vi "主页面.vi"() -> ()   [LabVIEW 2018]
uses:
  Global_Variable/A131258.vi
panel:
  out "8MPa正逆向差值":dbl format="%#.3g"
  out "压销力":bool
  out "内泄露":bool
  out "力特性":bool
  out "回正率":dbl format="%#.3g"
  out "右滞后最小值":dbl format="%#.3g"
  out "右滞后最大值":dbl format="%#.3g"
  out "左滞后最小值":dbl format="%#.3g"
  out "左滞后最大值":dbl format="%#.3g"
  out "力特性":cluster{dbl[], dbl[]}[](graph)
  out "布尔":bool
  out "压销力(N)":dbl format="%#.3g"
  out "右内泄露值(L)":dbl format="%#.3g"
  out "左内泄露值(L)":dbl format="%#.3g"
  out "1MPa逆向最大扭矩":dbl format="%#.3g"
  out "1MPa正向最大扭矩":dbl format="%#.3g"
  out "全曲线对称性":dbl format="%#.3g"
  out "5MPa对称性":dbl format="%#.3g"
  out "1MPa对称性":dbl format="%#.3g"
  out "8MPa逆向最大扭矩":dbl format="%#.3g"
  out "8MPa正向最大扭矩":dbl format="%#.3g"
  out "5MPa逆向最大扭矩":dbl format="%#.3g"
  out "5MPa正向最大扭矩":dbl format="%#.3g"
  out "3MPa逆向最大扭矩":dbl format="%#.3g"
  out "3MPa正向最大扭矩":dbl format="%#.3g"
  out "逆向最大油压":dbl format="%#.3g"
  out "正向最大油压":dbl format="%#.3g"
  out "逆向最大扭矩":dbl format="%#.3g"
  out "正向最大扭矩":dbl format="%#.3g"
  in  "停止":bool
  # "调阀台"
  # "-10    -9     -8     -7     -6      -5    -4      -3     -2     -1       0      1       2      3       4       5      6      7      8      9       10"
  # "9"
  # "8"
  # "7"
  # "6"
  # "5"
  # "4"
  # "3"
  # "2"
  # "1"
  # "0"
  # "-10    -9     -8     -7     -6      -5    -4      -3     -2     -1       0      1       2      3       4       5      6      7      8      9       10"
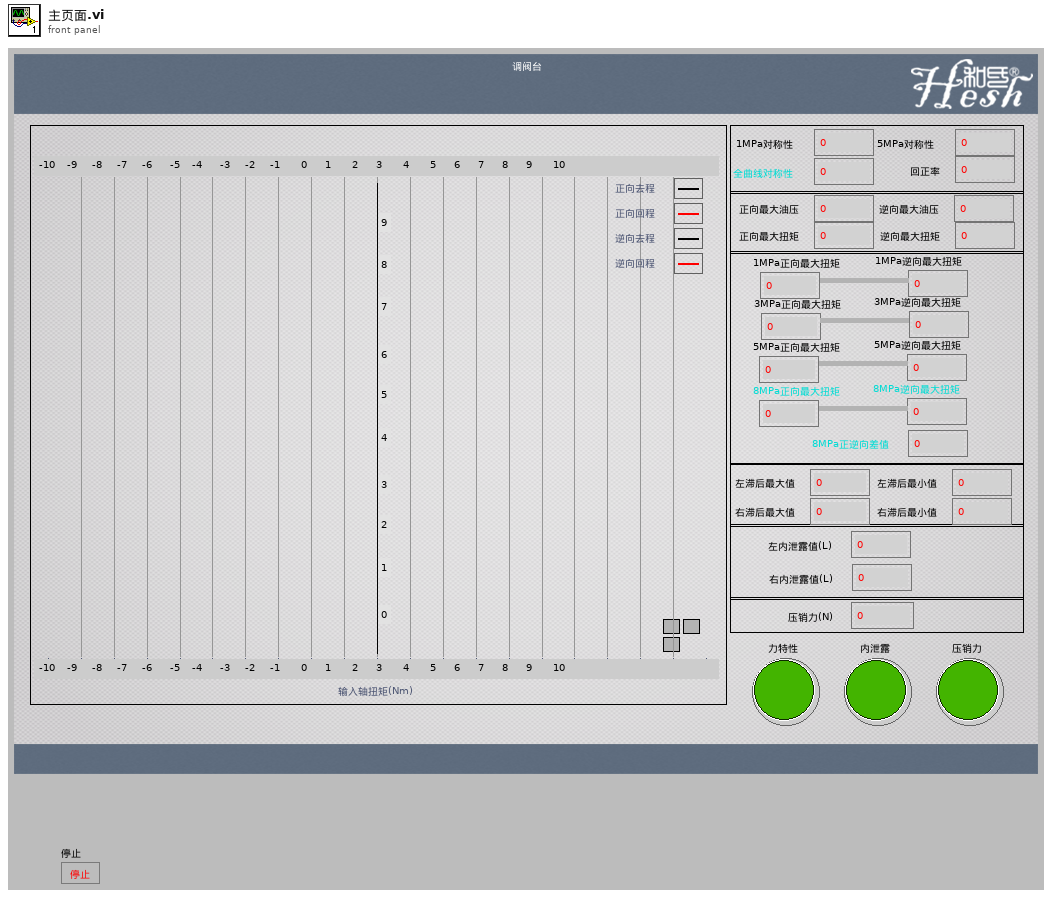
[diagram p1: front panel]
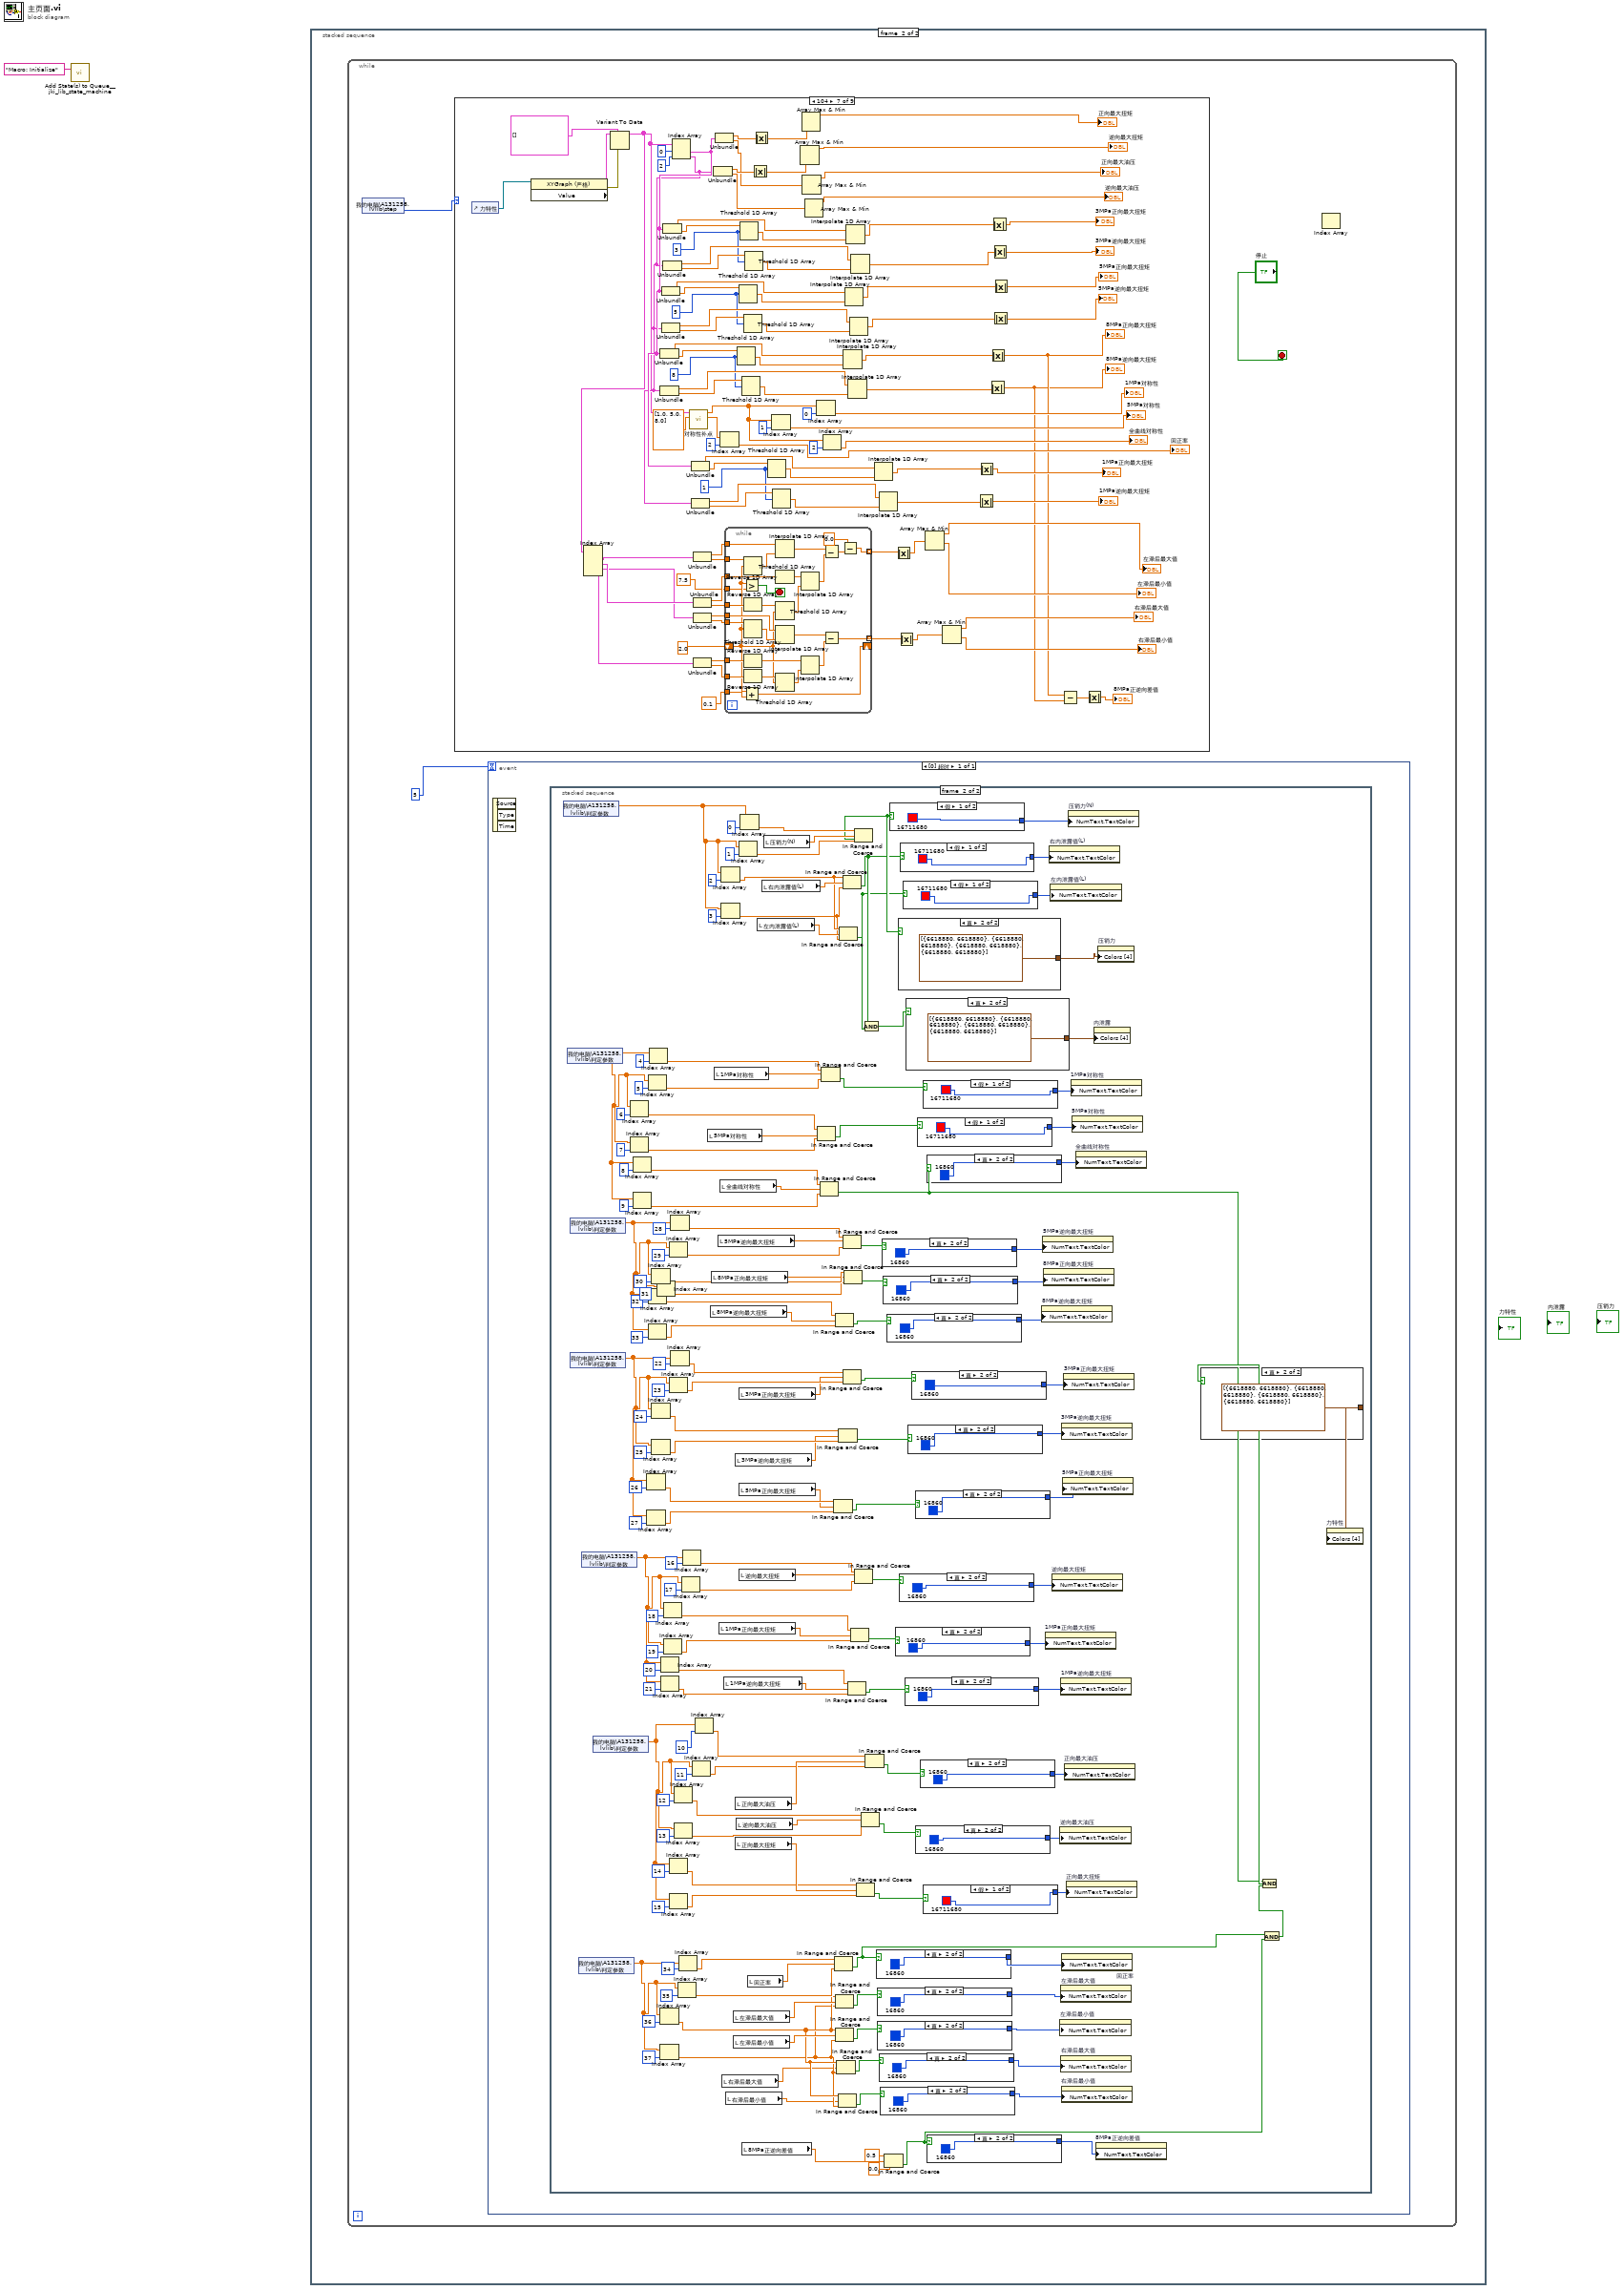
[diagram p0: block diagram]
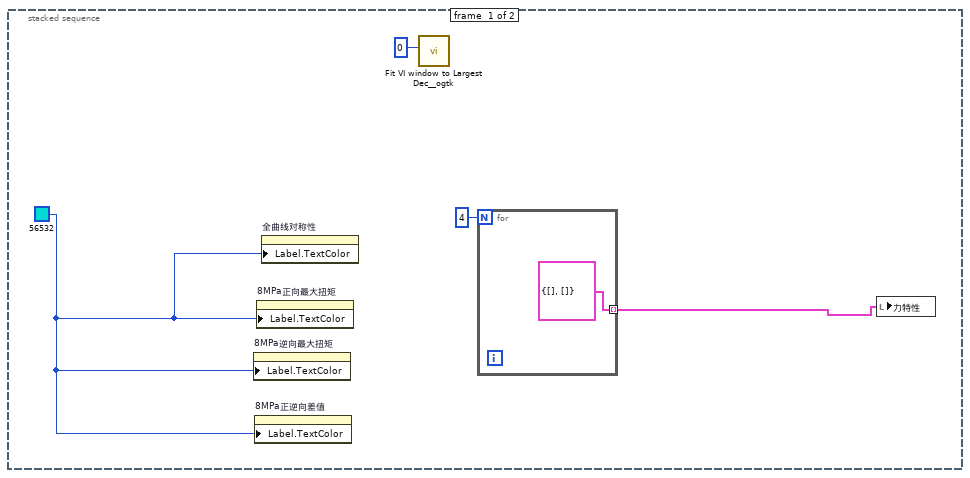
[diagram p2: hidden frame]
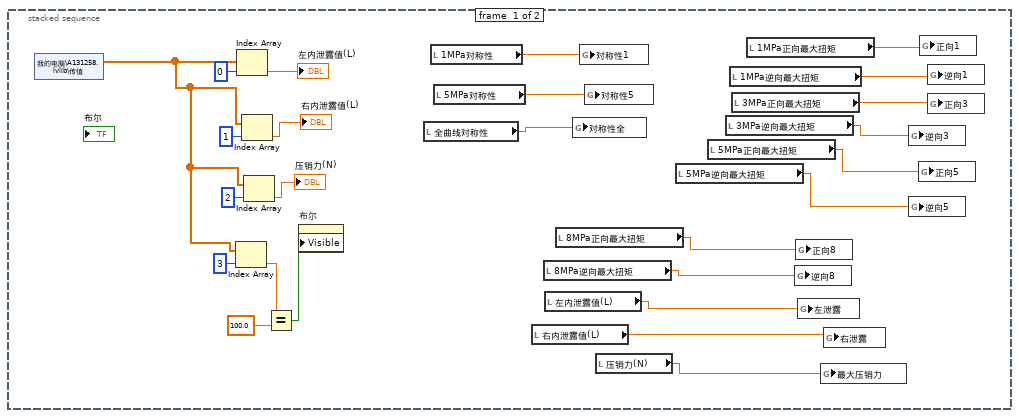
[diagram p3: hidden frame]
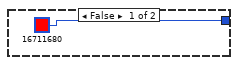
[diagram p4: hidden frame]
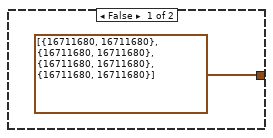
[diagram p5: hidden frame]
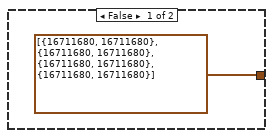
[diagram p6: hidden frame]
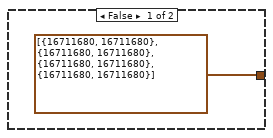
[diagram p7: hidden frame]
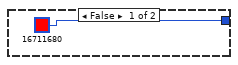
[diagram p8: hidden frame]
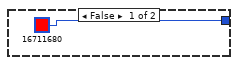
[diagram p9: hidden frame]
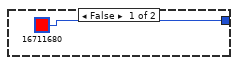
[diagram p10: hidden frame]
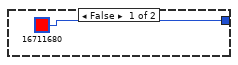
[diagram p11: hidden frame]
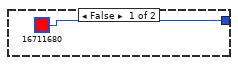
[diagram p12: hidden frame]
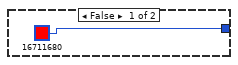
[diagram p13: hidden frame]
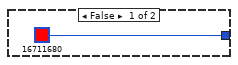
[diagram p14: hidden frame]
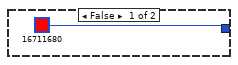
[diagram p15: hidden frame]
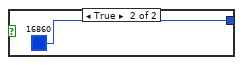
[diagram p16: hidden frame]
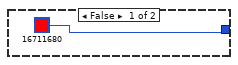
[diagram p17: hidden frame]
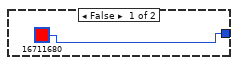
[diagram p18: hidden frame]
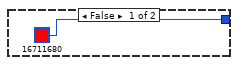
[diagram p19: hidden frame]
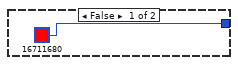
[diagram p20: hidden frame]
diagram:
  n1 = call <vilib>:"Add State(s) to Queue__jki_lib_state_machine.vi"("State(s) in (\"\")"="Macro: Initialize") -> ()  [unwired: 14 in, 1 out]
  n2 = stacked-sequence {
    frame #0 {
      w2 = u32 56532
      n3 = property on="8MPa逆向最大扭矩" class="DigNum (严格)"("Label.TextColor"=w2) -> ()  [unwired: 2 in, 2 out]
      n4 = property on="8MPa正逆向差值" class="DigNum (严格)"("Label.TextColor"=w2) -> ()  [unwired: 2 in, 2 out]
      n5 = property on="8MPa正向最大扭矩" class="DigNum (严格)"("Label.TextColor"=w2) -> ()  [unwired: 2 in, 2 out]
      n6 = property on="全曲线对称性" class="DigNum (严格)"("Label.TextColor"=w2) -> ()  [unwired: 2 in, 2 out]
      n7 = call <userlib>:"Fit VI window to Largest Dec__ogtk.vi"("border spacing (2 px)"=0) -> ()  [unwired: 5 in, 2 out]
      n8 = for {
        N: 4 -> [_]
        tunnel: [cluster{dbl[], dbl[]} {[], []}] -> w4 mode=indexing
      }
      n9 = local write "力特性"(w4) -> ()
    }
    frame #1 {
      n10 = while {
        stop <- "停止" stop-if-true
        n11 = shared-variable "我的电脑\\A131258.lvlib\\step"() -> (w8:u16)  [unwired: 1 in, 1 out]
        n12 = case shown="104" w8 {
          frame 0, Default {
          }
          frame 1 {
          }
          frame 100 {
            n13 = local read "力特性"() -> (w252:cluster{dbl[], dbl[]}[])
            n14 = for {
              tunnel: [w256] -> w253 mode=indexing
              tunnel: w252 -> [w255] mode=indexing
              i -> [w254]
              n15 = case shown="0" w254 {
                tunnel: [w257 w261] -> w256
                tunnel: w255 -> [w257 w260]
                frame Default {
                }
                frame 0 {
                  n16 = Unbundle(w260) -> (w265:dbl[], w264:dbl[])
                  n17 = shared-variable "我的电脑\\A131258.lvlib\\油压"() -> (w269:sgl[])  [unwired: 1 in, 1 out]
                  n18 = shared-variable "我的电脑\\A131258.lvlib\\扭力"() -> (w267:sgl[])  [unwired: 1 in, 1 out]
                  n19 = Index Array(array=w267, index=4) -> (element=w258:sgl)
                  n20 = Index Array(array=w269, index=4) -> (element=w259:sgl)
                  n21 = Build Array (concatenate)(w265, w258) -> (w263:dbl[])
                  n22 = Build Array (concatenate)(w264, w259) -> (w262:dbl[])
                  n23 = Bundle(w263, w262) -> (w261:cluster{dbl[], dbl[]})  [unwired: 1 in]
                }
              }
            }
            n24 = local write "力特性"(w253) -> ()
          }
          frame 101 {
            n25 = local read "力特性"() -> (w270:cluster{dbl[], dbl[]}[])
            n26 = for {
              tunnel: [w274] -> w271 mode=indexing
              tunnel: w270 -> [w273] mode=indexing
              i -> [w272]
              n27 = case shown="1" w272 {
                tunnel: [w275 w279] -> w274
                tunnel: w273 -> [w275 w278]
                frame Default {
                }
                frame 1 {
                  n28 = Unbundle(w278) -> (w283:dbl[], w282:dbl[])
                  n29 = shared-variable "我的电脑\\A131258.lvlib\\油压"() -> (w287:sgl[])  [unwired: 1 in, 1 out]
                  n30 = shared-variable "我的电脑\\A131258.lvlib\\扭力"() -> (w285:sgl[])  [unwired: 1 in, 1 out]
                  n31 = Index Array(array=w285, index=4) -> (element=w276:sgl)
                  n32 = Index Array(array=w287, index=4) -> (element=w277:sgl)
                  n33 = Build Array (concatenate)(w283, w276) -> (w281:dbl[])
                  n34 = Build Array (concatenate)(w282, w277) -> (w280:dbl[])
                  n35 = Bundle(w281, w280) -> (w279:cluster{dbl[], dbl[]})  [unwired: 1 in]
                }
              }
            }
            n36 = local write "力特性"(w271) -> ()
          }
          frame 102 {
            n37 = local read "力特性"() -> (w288:cluster{dbl[], dbl[]}[])
            n38 = for {
              tunnel: [w292] -> w289 mode=indexing
              tunnel: w288 -> [w291] mode=indexing
              i -> [w290]
              n39 = case shown="2" w290 {
                tunnel: [w293 w297] -> w292
                tunnel: w291 -> [w293 w296]
                frame Default {
                }
                frame 2 {
                  n40 = Unbundle(w296) -> (w301:dbl[], w300:dbl[])
                  n41 = shared-variable "我的电脑\\A131258.lvlib\\油压"() -> (w305:sgl[])  [unwired: 1 in, 1 out]
                  n42 = shared-variable "我的电脑\\A131258.lvlib\\扭力"() -> (w303:sgl[])  [unwired: 1 in, 1 out]
                  n43 = Index Array(array=w303, index=4) -> (element=w294:sgl)
                  n44 = Index Array(array=w305, index=4) -> (element=w295:sgl)
                  n45 = Build Array (concatenate)(w301, w294) -> (w299:dbl[])
                  n46 = Build Array (concatenate)(w300, w295) -> (w298:dbl[])
                  n47 = Bundle(w299, w298) -> (w297:cluster{dbl[], dbl[]})  [unwired: 1 in]
                }
              }
            }
            n48 = local write "力特性"(w289) -> ()
          }
          frame 103 {
            n49 = local read "力特性"() -> (w306:cluster{dbl[], dbl[]}[])
            n50 = for {
              tunnel: [w310] -> w307 mode=indexing
              tunnel: w306 -> [w309] mode=indexing
              i -> [w308]
              n51 = case shown="3" w308 {
                tunnel: [w311 w315] -> w310
                tunnel: w309 -> [w311 w314]
                frame Default {
                }
                frame 3 {
                  n52 = Unbundle(w314) -> (w319:dbl[], w318:dbl[])
                  n53 = shared-variable "我的电脑\\A131258.lvlib\\油压"() -> (w323:sgl[])  [unwired: 1 in, 1 out]
                  n54 = shared-variable "我的电脑\\A131258.lvlib\\扭力"() -> (w321:sgl[])  [unwired: 1 in, 1 out]
                  n55 = Index Array(array=w321, index=4) -> (element=w312:sgl)
                  n56 = Index Array(array=w323, index=4) -> (element=w313:sgl)
                  n57 = Build Array (concatenate)(w319, w312) -> (w317:dbl[])
                  n58 = Build Array (concatenate)(w318, w313) -> (w316:dbl[])
                  n59 = Bundle(w317, w316) -> (w315:cluster{dbl[], dbl[]})  [unwired: 1 in]
                }
              }
            }
            n60 = local write "力特性"(w307) -> ()
          }
          frame 104 {
            w381 = 1
            w388 = 8
            w395 = 5
            w402 = 3
            n61 = control-ref of="力特性"() -> (w355:refnum<vi>)
            n62 = property class="XYGraph (严格)"(reference=w355) -> (error out=w422:errorcluster, "Value"=w421:cluster{dbl[], dbl[]}[])  [unwired: 1 in, 1 out]
            n63 = Variant To Data(error in=w422, type=cluster{dbl[], dbl[]}[] [], Variant=w421) -> (data=w354:cluster{dbl[], dbl[]}[])  [unwired: 1 out]
            n64 = Index Array(array=w354) -> (element #1=w342:cluster{dbl[], dbl[]}, element #2=w341:cluster{dbl[], dbl[]}, element #3=w340:cluster{dbl[], dbl[]}, element #4=w339:cluster{dbl[], dbl[]})  [unwired: 4 in]
            n65 = Index Array(array=w354, index #1=0 ("索引"), index #2=2 ("索引")) -> (element #1=w379:cluster{dbl[], dbl[]}, element #2=w378:cluster{dbl[], dbl[]})
            n66 = Unbundle(w379) -> (w387:dbl[], w393:dbl[])
            n67 = Unbundle(w378) -> (w389:dbl[], w392:dbl[])
            n68 = Unbundle(w379) -> (w394:dbl[], w400:dbl[])
            n69 = Unbundle(w378) -> (w396:dbl[], w399:dbl[])
            n70 = Unbundle(w379) -> (w401:dbl[], w407:dbl[])
            n71 = Unbundle(w378) -> (w403:dbl[], w406:dbl[])
            n72 = call "对称性补点.vi"("检测点"=dbl[] [1.0, 5.0, 8.0], "XY图"=w354) -> ("回正率"=w329:dbl[], "对称性"=w375:dbl[])  [unwired: 8 in]
            n73 = Unbundle(w379) -> (w380:dbl[], w386:dbl[])
            n74 = Unbundle(w378) -> (w382:dbl[], w385:dbl[])
            n75 = Unbundle(w342) -> (w353:dbl[], w350:dbl[])
            n76 = Unbundle(w341) -> (w349:dbl[], w348:dbl[])
            n77 = Unbundle(w340) -> (w351:dbl[], w352:dbl[])
            n78 = Unbundle(w339) -> (w347:dbl[], w346:dbl[])
            n79 = Unbundle(w378) -> (w417:dbl[], w410:dbl[])
            n80 = Unbundle(w379) -> (w420:dbl[], w411:dbl[])
            n81 = Index Array(array=w329, index=2 ("索引")) -> (element=→"回正率":dbl)
            n82 = while {
              tunnel: w353 -> [w451]
              tunnel: w352 -> [w450]
              tunnel: w351 -> [w449]
              tunnel: w350 -> [w448]
              tunnel: w349 -> [w443]
              tunnel: w348 -> [w441]
              tunnel: w347 -> [w439]
              tunnel: w346 -> [w437]
              tunnel: [w424] -> w334 mode=indexing
              tunnel: [w423] -> w332 mode=indexing
              shift-right: [w430] -> _
              shift-left: 2.0 ("精度") -> [w429]
              tunnel: 0.1 ("精度") -> [w431]
              tunnel: 7.5 ("精度") -> [w428]
              stop <- w427 stop-if-true
              n83 = Greater?(x=w429, y=w428) -> (0:w427:bool)
              n84 = Add(x=w429, y=w431) -> (x+y=w430:dbl)
              n85 = Threshold 1D Array(2:w429, 3:w448) -> (0:w447:dbl)  [unwired: 1 in]
              n86 = Reverse 1D Array(array=w441) -> (reversed array=w440:dbl[])
              n87 = Threshold 1D Array(2:w429, 3:w450) -> (0:w446:dbl)  [unwired: 1 in]
              n88 = Reverse 1D Array(array=w439) -> (reversed array=w438:dbl[])
              n89 = Reverse 1D Array(array=w437) -> (reversed array=w436:dbl[])
              n90 = Interpolate 1D Array(1:w447, 2:w451) -> (0:w435:dbl)
              n91 = Reverse 1D Array(array=w443) -> (reversed array=w442:dbl[])
              n92 = Threshold 1D Array(2:w429, 3:w440) -> (0:w445:dbl)  [unwired: 1 in]
              n93 = Interpolate 1D Array(1:w446, 2:w449) -> (0:w433:dbl)
              n94 = Threshold 1D Array(2:w429, 3:w436) -> (0:w444:dbl)  [unwired: 1 in]
              n95 = Interpolate 1D Array(1:w445, 2:w442) -> (0:w434:dbl)
              n96 = Interpolate 1D Array(1:w444, 2:w438) -> (0:w432:dbl)
              n97 = Subtract(x=w435, y=w434) -> (x-y=w426:dbl)
              n98 = Subtract(x=w433, y=w432) -> (x-y=w423:dbl)
              n99 = Subtract(x=0.0, y=w426) -> (x-y=w424:dbl)
            }
            n100 = Threshold 1D Array(2:w388, 3:w393) -> (0:w391:dbl)  [unwired: 1 in]
            n101 = Threshold 1D Array(2:w395, 3:w400) -> (0:w398:dbl)  [unwired: 1 in]
            n102 = Threshold 1D Array(2:w402, 3:w407) -> (0:w405:dbl)  [unwired: 1 in]
            n103 = Threshold 1D Array(2:w388, 3:w392) -> (0:w390:dbl)  [unwired: 1 in]
            n104 = Threshold 1D Array(2:w395, 3:w399) -> (0:w397:dbl)  [unwired: 1 in]
            n105 = Threshold 1D Array(2:w402, 3:w406) -> (0:w404:dbl)  [unwired: 1 in]
            n106 = Absolute Value(x=w417) -> (abs(x)=w416:dbl[])
            n107 = Absolute Value(x=w420) -> (abs(x)=w419:dbl[])
            n108 = Threshold 1D Array(2:w381, 3:w386) -> (0:w384:dbl)  [unwired: 1 in]
            n109 = Index Array(array=w375, index=1 ("索引")) -> (element=→"5MPa对称性":dbl)
            n110 = Threshold 1D Array(2:w381, 3:w385) -> (0:w383:dbl)  [unwired: 1 in]
            n111 = Array Max & Min(array=w416) -> (max value=→"逆向最大扭矩":dbl)  [unwired: 3 out]
            n112 = Array Max & Min(array=w419) -> (max value=→"正向最大扭矩":dbl)  [unwired: 3 out]
            n113 = Array Max & Min(array=w411) -> (max value=→"正向最大油压":dbl)  [unwired: 3 out]
            n114 = Array Max & Min(array=w410) -> (max value=→"逆向最大油压":dbl)  [unwired: 3 out]
            n115 = Index Array(array=w375, index=0 ("索引")) -> (element=→"1MPa对称性":dbl)
            n116 = Index Array(array=w375, index=2 ("索引")) -> (element=→"全曲线对称性":dbl)
            n117 = Interpolate 1D Array(1:w391, 2:w387) -> (0:w361:dbl)
            n118 = Interpolate 1D Array(1:w398, 2:w394) -> (0:w365:dbl)
            n119 = Interpolate 1D Array(1:w405, 2:w401) -> (0:w369:dbl)
            n120 = Interpolate 1D Array(1:w390, 2:w389) -> (0:w360:dbl)
            n121 = Interpolate 1D Array(1:w397, 2:w396) -> (0:w362:dbl)
            n122 = Interpolate 1D Array(1:w404, 2:w403) -> (0:w367:dbl)
            n123 = Interpolate 1D Array(1:w384, 2:w380) -> (0:w359:dbl)
            n124 = Interpolate 1D Array(1:w383, 2:w382) -> (0:w357:dbl)
            n125 = Absolute Value(x=w334) -> (abs(x)=w333:dbl[])
            n126 = Absolute Value(x=w332) -> (abs(x)=w331:dbl[])
            n127 = Array Max & Min(array=w333) -> (max value=→"左滞后最大值":dbl, min value=→"左滞后最小值":dbl)  [unwired: 2 out]
            n128 = Array Max & Min(array=w331) -> (max value=→"右滞后最大值":dbl, min value=→"右滞后最小值":dbl)  [unwired: 2 out]
            n129 = Absolute Value(x=w357) -> (abs(x)=→"1MPa逆向最大扭矩":dbl)
            n130 = Absolute Value(x=w359) -> (abs(x)=→"1MPa正向最大扭矩":dbl)
            n131 = Absolute Value(x=w360) -> (abs(x)=w324:dbl)
            "8MPa逆向最大扭矩" <- w324
            n132 = Absolute Value(x=w361) -> (abs(x)=w325:dbl)
            "8MPa正向最大扭矩" <- w325
            n133 = Absolute Value(x=w369) -> (abs(x)=→"3MPa正向最大扭矩":dbl)
            n134 = Absolute Value(x=w367) -> (abs(x)=→"3MPa逆向最大扭矩":dbl)
            n135 = Absolute Value(x=w362) -> (abs(x)=→"5MPa逆向最大扭矩":dbl)
            n136 = Absolute Value(x=w365) -> (abs(x)=→"5MPa正向最大扭矩":dbl)
            n137 = Subtract(x=w325, y=w324) -> (x-y=w327:dbl)
            n138 = Absolute Value(x=w327) -> (abs(x)=→"8MPa正逆向差值":dbl)
          }
          frame 105 {
            n139 = for {
              N: 4 -> [_]
              tunnel: [cluster{dbl[], dbl[]} {[], []}] -> w452 mode=indexing
            }
            "力特性" <- w452
          }
          frame 106 {
            n140 = control-ref of="力特性"() -> (w455:refnum<vi>)
            n141 = global write "A131258.vi" "力特性曲线"(w455) -> ()
            n142 = call "Report.vi"() -> ()  [unwired: 11 in, 1 out]
          }
        }
        n143 = event shown="[0] 超时" {
          selector: _ -> [_]
          dyn-events: _ -> [_]
          timeout: 5 -> [_]
          event Timeout {
            n144 = event-data() -> ()  [unwired: 1 in, 3 out]
            n145 = stacked-sequence {
              frame #0 {
                n146 = shared-variable "我的电脑\\A131258.lvlib\\传值"() -> (w32:sgl[])  [unwired: 1 in, 1 out]
                n147 = Index Array(array=w32, index=3 ("索引")) -> (element=w33:sgl)
                n148 = Index Array(array=w32, index=0 ("索引")) -> (element=→"左内泄露值(L)":sgl)
                n149 = Index Array(array=w32, index=1 ("索引")) -> (element=→"右内泄露值(L)":sgl)
                n150 = Index Array(array=w32, index=2 ("索引")) -> (element=→"压销力(N)":sgl)
                n151 = Equal?(x=w33, y=sgl 100.0) -> (x = y?=w34:bool)
                n152 = property on="布尔" class="Bool (严格)"("Visible"=w34) -> ()  [unwired: 2 in, 2 out]
                n153 = local read "全曲线对称性"() -> (w21:dbl)
                n154 = local read "1MPa对称性"() -> (w23:dbl)
                n155 = local read "5MPa对称性"() -> (w22:dbl)
                n156 = local read "右内泄露值(L)"() -> (w13:dbl)
                n157 = local read "8MPa逆向最大扭矩"() -> (w11:dbl)
                n158 = local read "左内泄露值(L)"() -> (w12:dbl)
                n159 = local read "8MPa正向最大扭矩"() -> (w10:dbl)
                n160 = global write "A131258.vi" "对称性全"(w21) -> ()
                n161 = global write "A131258.vi" "对称性1"(w23) -> ()
                n162 = global write "A131258.vi" "对称性5"(w22) -> ()
                n163 = local read "压销力(N)"() -> (w14:dbl)
                n164 = local read "5MPa逆向最大扭矩"() -> (w20:dbl)
                n165 = local read "5MPa正向最大扭矩"() -> (w19:dbl)
                n166 = local read "3MPa逆向最大扭矩"() -> (w18:dbl)
                n167 = local read "1MPa逆向最大扭矩"() -> (w16:dbl)
                n168 = local read "3MPa正向最大扭矩"() -> (w17:dbl)
                n169 = local read "1MPa正向最大扭矩"() -> (w15:dbl)
                n170 = global write "A131258.vi" "逆向8"(w11) -> ()
                n171 = global write "A131258.vi" "正向8"(w10) -> ()
                n172 = global write "A131258.vi" "左泄露"(w12) -> ()
                n173 = global write "A131258.vi" "最大压销力"(w14) -> ()
                n174 = global write "A131258.vi" "右泄露"(w13) -> ()
                n175 = global write "A131258.vi" "逆向3"(w18) -> ()
                n176 = global write "A131258.vi" "逆向5"(w20) -> ()
                n177 = global write "A131258.vi" "正向5"(w19) -> ()
                n178 = global write "A131258.vi" "正向1"(w15) -> ()
                n179 = global write "A131258.vi" "逆向1"(w16) -> ()
                n180 = global write "A131258.vi" "正向3"(w17) -> ()
              }
              frame #1 {
                n181 = shared-variable "我的电脑\\A131258.lvlib\\判定参数"() -> (w188:sgl[])  [unwired: 1 in, 1 out]
                n182 = shared-variable "我的电脑\\A131258.lvlib\\判定参数"() -> (w185:sgl[])  [unwired: 1 in, 1 out]
                n183 = shared-variable "我的电脑\\A131258.lvlib\\判定参数"() -> (w167:sgl[])  [unwired: 1 in, 1 out]
                n184 = shared-variable "我的电脑\\A131258.lvlib\\判定参数"() -> (w145:sgl[])  [unwired: 1 in, 1 out]
                n185 = shared-variable "我的电脑\\A131258.lvlib\\判定参数"() -> (w83:sgl[])  [unwired: 1 in, 1 out]
                n186 = shared-variable "我的电脑\\A131258.lvlib\\判定参数"() -> (w123:sgl[])  [unwired: 1 in, 1 out]
                n187 = shared-variable "我的电脑\\A131258.lvlib\\判定参数"() -> (w108:sgl[])  [unwired: 1 in, 1 out]
                n188 = Index Array(array=w185, index=6 ("索引")) -> (element=w179:sgl)
                n189 = Index Array(array=w185, index=7 ("索引")) -> (element=w177:sgl)
                n190 = Index Array(array=w185, index=8 ("索引")) -> (element=w176:sgl)
                n191 = Index Array(array=w185, index=9 ("索引")) -> (element=w174:sgl)
                n192 = Index Array(array=w145, index=26 ("索引")) -> (element=w137:sgl)
                n193 = Index Array(array=w145, index=27 ("索引")) -> (element=w136:sgl)
                n194 = Index Array(array=w185, index=5 ("索引")) -> (element=w182:sgl)
                n195 = Index Array(array=w167, index=32 ("索引")) -> (element=w154:sgl)
                n196 = Index Array(array=w167, index=33 ("索引")) -> (element=w152:sgl)
                n197 = Index Array(array=w185, index=4 ("索引")) -> (element=w184:sgl)
                n198 = Index Array(array=w167, index=30 ("索引")) -> (element=w157:sgl)
                n199 = Index Array(array=w145, index=24 ("索引")) -> (element=w139:sgl)
                n200 = Index Array(array=w145, index=25 ("索引")) -> (element=w138:sgl)
                n201 = Index Array(array=w167, index=31 ("索引")) -> (element=w155:sgl)
                n202 = Index Array(array=w83, index=36 ("索引")) -> (element=w63:sgl)
                n203 = Index Array(array=w83, index=37 ("索引")) -> (element=w62:sgl)
                n204 = Index Array(array=w123, index=20 ("索引")) -> (element=w114:sgl)
                n205 = Index Array(array=w123, index=21 ("索引")) -> (element=w113:sgl)
                n206 = Index Array(array=w123, index=18 ("索引")) -> (element=w116:sgl)
                n207 = Index Array(array=w123, index=19 ("索引")) -> (element=w115:sgl)
                n208 = Index Array(array=w167, index=29 ("索引")) -> (element=w161:sgl)
                n209 = Index Array(array=w145, index=23 ("索引")) -> (element=w140:sgl)
                n210 = Index Array(array=w108, index=14 ("索引")) -> (element=w100:sgl)
                n211 = Index Array(array=w108, index=15 ("索引")) -> (element=w99:sgl)
                n212 = Index Array(array=w167, index=28 ("索引")) -> (element=w163:sgl)
                n213 = Index Array(array=w145, index=22 ("索引")) -> (element=w141:sgl)
                n214 = Index Array(array=w108, index=12 ("索引")) -> (element=w102:sgl)
                n215 = Index Array(array=w108, index=13 ("索引")) -> (element=w101:sgl)
                n216 = Index Array(array=w83, index=35 ("索引")) -> (element=w75:sgl)
                n217 = Index Array(array=w83, index=34 ("索引")) -> (element=w77:sgl)
                n218 = Index Array(array=w123, index=17 ("索引")) -> (element=w120:sgl)
                n219 = Index Array(array=w123, index=16 ("索引")) -> (element=w121:sgl)
                n220 = Index Array(array=w108, index=11 ("索引")) -> (element=w103:sgl)
                n221 = Index Array(array=w108, index=10 ("索引")) -> (element=w104:sgl)
                n222 = local read "5MPa对称性"() -> (w178:dbl)
                n223 = local read "8MPa逆向最大扭矩"() -> (w153:dbl)
                n224 = local read "8MPa正向最大扭矩"() -> (w156:dbl)
                n225 = local read "1MPa对称性"() -> (w183:dbl)
                n226 = local read "5MPa逆向最大扭矩"() -> (w162:dbl)
                n227 = local read "1MPa正向最大扭矩"() -> (w118:dbl)
                n228 = local read "全曲线对称性"() -> (w175:dbl)
                n229 = Index Array(array=w188, index=2 ("索引")) -> (element=w187:sgl)
                n230 = Index Array(array=w188, index=3 ("索引")) -> (element=w186:sgl)
                n231 = local read "右滞后最大值"() -> (w61:dbl)
                n232 = local read "1MPa逆向最大扭矩"() -> (w117:dbl)
                n233 = local read "右滞后最小值"() -> (w60:dbl)
                n234 = local read "左滞后最大值"() -> (w65:dbl)
                n235 = local read "左滞后最小值"() -> (w64:dbl)
                n236 = local read "3MPa逆向最大扭矩"() -> (w134:dbl)
                n237 = local read "正向最大油压"() -> (w107:dbl)
                n238 = local read "正向最大扭矩"() -> (w105:dbl)
                n239 = local read "逆向最大油压"() -> (w106:dbl)
                n240 = Index Array(array=w188, index=1 ("索引")) -> (element=w196:sgl)
                n241 = local read "3MPa正向最大扭矩"() -> (w135:dbl)
                n242 = local read "5MPa正向最大扭矩"() -> (w133:dbl)
                n243 = local read "逆向最大扭矩"() -> (w122:dbl)
                n244 = Index Array(array=w188, index=0 ("索引")) -> (element=w197:sgl)
                n245 = local read "8MPa正逆向差值"() -> (w40:dbl)
                n246 = local read "回正率"() -> (w76:dbl)
                n247 = local read "左内泄露值(L)"() -> (w189:dbl)
                n248 = local read "右内泄露值(L)"() -> (w190:dbl)
                n249 = local read "压销力(N)"() -> (w195:dbl)
                n250 = In Range and Coerce(upper limit=w179, x=w178, lower limit=w177) -> (In Range?=w180:bool)  [unwired: 1 out]
                n251 = In Range and Coerce(upper limit=w176, x=w175, lower limit=w174) -> (In Range?=w42:bool)  [unwired: 1 out]
                n252 = In Range and Coerce(upper limit=w184, x=w183, lower limit=w182) -> (In Range?=w181:bool)  [unwired: 1 out]
                n253 = In Range and Coerce(upper limit=w137, x=w133, lower limit=w136) -> (In Range?=w142:bool)  [unwired: 1 out]
                n254 = In Range and Coerce(upper limit=w77, x=w76, lower limit=w75) -> (In Range?=w37:bool)  [unwired: 1 out]
                n255 = In Range and Coerce(upper limit=w154, x=w153, lower limit=w152) -> (In Range?=w158:bool)  [unwired: 1 out]
                n256 = In Range and Coerce(upper limit=w63, x=w65, lower limit=w62) -> (In Range?=w73:bool)  [unwired: 1 out]
                n257 = In Range and Coerce(upper limit=w63, x=w64, lower limit=w62) -> (In Range?=w72:bool)  [unwired: 1 out]
                n258 = In Range and Coerce(upper limit=w63, x=w61, lower limit=w62) -> (In Range?=w71:bool)  [unwired: 1 out]
                n259 = In Range and Coerce(upper limit=w63, x=w60, lower limit=w62) -> (In Range?=w70:bool)  [unwired: 1 out]
                n260 = In Range and Coerce(upper limit=w139, x=w134, lower limit=w138) -> (In Range?=w143:bool)  [unwired: 1 out]
                n261 = In Range and Coerce(upper limit=w187, x=w189, lower limit=w186) -> (In Range?=w45:bool)  [unwired: 1 out]
                n262 = In Range and Coerce(upper limit=w187, x=w190, lower limit=w186) -> (In Range?=w46:bool)  [unwired: 1 out]
                n263 = In Range and Coerce(upper limit=w163, x=w162, lower limit=w161) -> (In Range?=w160:bool)  [unwired: 1 out]
                n264 = In Range and Coerce(upper limit=w141, x=w135, lower limit=w140) -> (In Range?=w144:bool)  [unwired: 1 out]
                n265 = In Range and Coerce(upper limit=w157, x=w156, lower limit=w155) -> (In Range?=w159:bool)  [unwired: 1 out]
                n266 = In Range and Coerce(upper limit=w114, x=w117, lower limit=w113) -> (In Range?=w111:bool)  [unwired: 1 out]
                n267 = In Range and Coerce(upper limit=w116, x=w118, lower limit=w115) -> (In Range?=w112:bool)  [unwired: 1 out]
                n268 = In Range and Coerce(upper limit=w197, x=w195, lower limit=w196) -> (In Range?=w49:bool)  [unwired: 1 out]
                n269 = In Range and Coerce(upper limit=w121, x=w122, lower limit=w120) -> (In Range?=w119:bool)  [unwired: 1 out]
                n270 = In Range and Coerce(upper limit=w100, x=w105, lower limit=w99) -> (In Range?=w96:bool)  [unwired: 1 out]
                n271 = In Range and Coerce(upper limit=w102, x=w106, lower limit=w101) -> (In Range?=w97:bool)  [unwired: 1 out]
                n272 = And(x=w46, y=w45) -> (x .and. y?=w47:bool)
                n273 = In Range and Coerce(upper limit=w104, x=w107, lower limit=w103) -> (In Range?=w98:bool)  [unwired: 1 out]
                n274 = case shown="真" w37 {
                  tunnel: [u32 16711680 u32 16860] -> w74
                  frame False {
                  }
                  frame True {
                  }
                }
                n275 = case shown="真" w73 {
                  tunnel: [u32 16711680 u32 16860] -> w69
                  frame False {
                  }
                  frame True {
                  }
                }
                n276 = case shown="真" w72 {
                  tunnel: [u32 16711680 u32 16860] -> w68
                  frame False {
                  }
                  frame True {
                  }
                }
                n277 = case shown="真" w71 {
                  tunnel: [u32 16711680 u32 16860] -> w67
                  frame False {
                  }
                  frame True {
                  }
                }
                n278 = case shown="真" w70 {
                  tunnel: [u32 16711680 u32 16860] -> w66
                  frame False {
                  }
                  frame True {
                  }
                }
                n279 = case shown="真" w160 {
                  tunnel: [u32 16711680 u32 16860] -> w166
                  frame False {
                  }
                  frame True {
                  }
                }
                n280 = case shown="真" w159 {
                  tunnel: [u32 16711680 u32 16860] -> w165
                  frame False {
                  }
                  frame True {
                  }
                }
                n281 = In Range and Coerce(upper limit=0.5 ("上限"), x=w40, lower limit=0.0 ("下限")) -> (In Range?=w36:bool)  [unwired: 1 out]
                n282 = case shown="真" w158 {
                  tunnel: [u32 16711680 u32 16860] -> w164
                  frame False {
                  }
                  frame True {
                  }
                }
                n283 = case shown="假" w49 {
                  tunnel: [u32 16711680 u32 16860] -> w51
                  frame False {
                  }
                  frame True {
                  }
                }
                n284 = case shown="真" w112 {
                  tunnel: [u32 16711680 u32 16860] -> w110
                  frame False {
                  }
                  frame True {
                  }
                }
                n285 = case shown="真" w49 {
                  tunnel: [cluster{u32, u32}[] [{16711680, 16711680}, {16711680, 16711680}, {16711680, 16711680}, {16711680, 16711680}] cluster{u32, u32}[] [{6618880, 6618880}, {6618880, 6618880}, {6618880, 6618880}, {6618880, 6618880}]] -> w50
                  frame False {
                  }
                  frame True {
                  }
                }
                n286 = case shown="真" w119 {
                  tunnel: [u32 16711680 u32 16860] -> w78
                  frame False {
                  }
                  frame True {
                  }
                }
                n287 = case shown="假" w46 {
                  tunnel: [u32 16711680 u32 16860] -> w52
                  frame False {
                  }
                  frame True {
                  }
                }
                n288 = case shown="假" w45 {
                  tunnel: [u32 16711680 u32 16860] -> w53
                  frame False {
                  }
                  frame True {
                  }
                }
                n289 = case shown="真" w111 {
                  tunnel: [u32 16711680 u32 16860] -> w109
                  frame False {
                  }
                  frame True {
                  }
                }
                n290 = case shown="真" w47 {
                  tunnel: [cluster{u32, u32}[] [{16711680, 16711680}, {16711680, 16711680}, {16711680, 16711680}, {16711680, 16711680}] cluster{u32, u32}[] [{6618880, 6618880}, {6618880, 6618880}, {6618880, 6618880}, {6618880, 6618880}]] -> w48
                  frame False {
                  }
                  frame True {
                  }
                }
                n291 = case shown="真" w143 {
                  tunnel: [u32 16711680 u32 16860] -> w131
                  frame False {
                  }
                  frame True {
                  }
                }
                n292 = case shown="真" w144 {
                  tunnel: [u32 16711680 u32 16860] -> w132
                  frame False {
                  }
                  frame True {
                  }
                }
                n293 = case shown="真" w142 {
                  tunnel: [u32 16711680 u32 16860] -> w130
                  frame False {
                  }
                  frame True {
                  }
                }
                n294 = case shown="真" w97 {
                  tunnel: [u32 16711680 u32 16860] -> w58
                  frame False {
                  }
                  frame True {
                  }
                }
                n295 = case shown="假" w180 {
                  tunnel: [u32 16711680 u32 16860] -> w55
                  frame False {
                  }
                  frame True {
                  }
                }
                n296 = case shown="真" w98 {
                  tunnel: [u32 16711680 u32 16860] -> w59
                  frame False {
                  }
                  frame True {
                  }
                }
                n297 = case shown="假" w181 {
                  tunnel: [u32 16711680 u32 16860] -> w54
                  frame False {
                  }
                  frame True {
                  }
                }
                n298 = case shown="假" w96 {
                  tunnel: [u32 16711680 u32 16860] -> w57
                  frame False {
                  }
                  frame True {
                  }
                }
                n299 = case shown="真" w42 {
                  tunnel: [u32 16711680 u32 16860] -> w56
                  frame False {
                  }
                  frame True {
                  }
                }
                n300 = case shown="真" w36 {
                  tunnel: [u32 16711680 u32 16860] -> w41
                  frame False {
                  }
                  frame True {
                  }
                }
                n301 = property on="8MPa逆向最大扭矩" class="DigNum (严格)"("NumText.TextColor"=w164) -> ()  [unwired: 2 in, 2 out]
                n302 = property on="5MPa逆向最大扭矩" class="DigNum (严格)"("NumText.TextColor"=w166) -> ()  [unwired: 2 in, 2 out]
                n303 = property on="8MPa正向最大扭矩" class="DigNum (严格)"("NumText.TextColor"=w165) -> ()  [unwired: 2 in, 2 out]
                n304 = property on="1MPa正向最大扭矩" class="DigNum (严格)"("NumText.TextColor"=w110) -> ()  [unwired: 2 in, 2 out]
                n305 = property on="右内泄露值(L)" class="DigNum (严格)"("NumText.TextColor"=w52) -> ()  [unwired: 2 in, 2 out]
                n306 = property on="左内泄露值(L)" class="DigNum (严格)"("NumText.TextColor"=w53) -> ()  [unwired: 2 in, 2 out]
                n307 = property on="逆向最大扭矩" class="DigNum (严格)"("NumText.TextColor"=w78) -> ()  [unwired: 2 in, 2 out]
                n308 = property on="逆向最大油压" class="DigNum (严格)"("NumText.TextColor"=w58) -> ()  [unwired: 2 in, 2 out]
                n309 = property on="左滞后最小值" class="DigNum (严格)"("NumText.TextColor"=w68) -> ()  [unwired: 2 in, 2 out]
                n310 = property on="1MPa逆向最大扭矩" class="DigNum (严格)"("NumText.TextColor"=w109) -> ()  [unwired: 2 in, 2 out]
                n311 = property on="左滞后最大值" class="DigNum (严格)"("NumText.TextColor"=w69) -> ()  [unwired: 2 in, 2 out]
                n312 = property on="右滞后最大值" class="DigNum (严格)"("NumText.TextColor"=w67) -> ()  [unwired: 2 in, 2 out]
                n313 = property on="3MPa逆向最大扭矩" class="DigNum (严格)"("NumText.TextColor"=w131) -> ()  [unwired: 2 in, 2 out]
                n314 = property on="回正率" class="DigNum (严格)"("NumText.TextColor"=w74) -> ()  [unwired: 2 in, 2 out]
                n315 = property on="右滞后最小值" class="DigNum (严格)"("NumText.TextColor"=w66) -> ()  [unwired: 2 in, 2 out]
                n316 = property on="5MPa正向最大扭矩" class="DigNum (严格)"("NumText.TextColor"=w130) -> ()  [unwired: 2 in, 2 out]
                n317 = property on="3MPa正向最大扭矩" class="DigNum (严格)"("NumText.TextColor"=w132) -> ()  [unwired: 2 in, 2 out]
                n318 = property on="正向最大油压" class="DigNum (严格)"("NumText.TextColor"=w59) -> ()  [unwired: 2 in, 2 out]
                n319 = property on="正向最大扭矩" class="DigNum (严格)"("NumText.TextColor"=w57) -> ()  [unwired: 2 in, 2 out]
                n320 = property on="压销力(N)" class="DigNum (严格)"("NumText.TextColor"=w51) -> ()  [unwired: 2 in, 2 out]
                n321 = property on="1MPa对称性" class="DigNum (严格)"("NumText.TextColor"=w54) -> ()  [unwired: 2 in, 2 out]
                n322 = property on="5MPa对称性" class="DigNum (严格)"("NumText.TextColor"=w55) -> ()  [unwired: 2 in, 2 out]
                n323 = property on="全曲线对称性" class="DigNum (严格)"("NumText.TextColor"=w56) -> ()  [unwired: 2 in, 2 out]
                n324 = property on="内泄露" class="Bool (严格)"("Colors [4]"=w48) -> ()  [unwired: 2 in, 2 out]
                n325 = property on="8MPa正逆向差值" class="DigNum (严格)"("NumText.TextColor"=w41) -> ()  [unwired: 2 in, 2 out]
                n326 = property on="压销力" class="Bool (严格)"("Colors [4]"=w50) -> ()  [unwired: 2 in, 2 out]
                n327 = And(x=w37, y=w36) -> (x .and. y?=w35:bool)
                n328 = And(x=w42, y=w35) -> (x .and. y?=w43:bool)
                n329 = case shown="真" w43 {
                  tunnel: [cluster{u32, u32}[] [{16711680, 16711680}, {16711680, 16711680}, {16711680, 16711680}, {16711680, 16711680}] cluster{u32, u32}[] [{6618880, 6618880}, {6618880, 6618880}, {6618880, 6618880}, {6618880, 6618880}]] -> w44
                  frame False {
                  }
                  frame True {
                  }
                }
                n330 = property on="力特性" class="Bool (严格)"("Colors [4]"=w44) -> ()  [unwired: 2 in, 2 out]
              }
            }
          }
        }
        n331 = Index Array() -> ()  [unwired: 2 in, 1 out]
      }
    }
  }
